vi "Open Sample Container Connections.vi"(8 "error in (no error)":errorcluster, 11 "Sample Line in":refnum<class "Sample Line.lvclass">) -> (0 "error out":errorcluster, 3 "Sample Line out":refnum<class "Sample Line.lvclass">)   [LabVIEW 2015, in "cRIO-Carbondioxide.lvlib" / "CO2-Actor.lvlib" / "Sample Line.lvclass"]
uses:
  Sample Line.lvclass
  Sample Line.lvclass/Sample Line.ctl
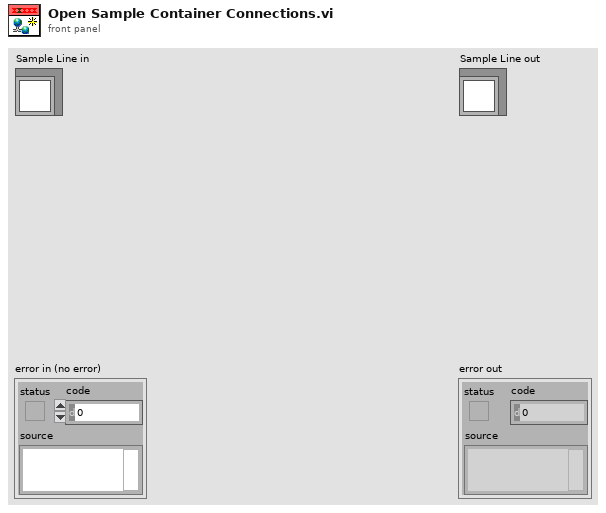
[diagram p1: front panel]
types:
  T1 = typedef "Sample Container.ctl" = cluster{"Sample In":refnum<k21>, "Sample Name":refnum<k21>, "Ti Cathode":refnum<k21>, "SampleQ":refnum<queue>}
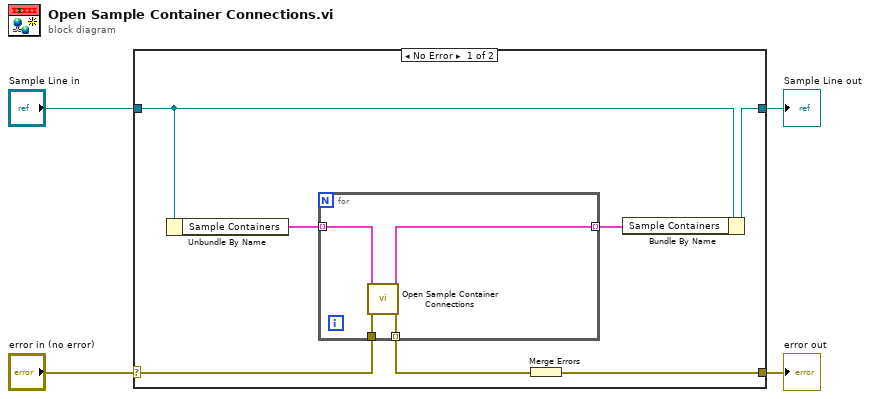
[diagram p0: block diagram]
diagram:
  n1 = case shown="No Error" "error in (no error)" {
    selector: "error in (no error)" -> [w10 w17]
    tunnel: [w8 w17] -> w3
    tunnel: [w5 w16] -> w1
    tunnel: "Sample Line in" -> [w6 w16]
    frame No Error {
      n2 = Unbundle By Name(w6) -> ("Sample Containers"=w11:T1[])
      n3 = for {
        tunnel: w11 -> [w14] mode=indexing
        tunnel: w10 -> [w15]
        tunnel: [w13] -> w7 mode=indexing
        tunnel: [w12] -> w9 mode=indexing
        n4 = call "Open Sample Container Connections.vi"("error in (no error)"=w15, "Container in"=w14) -> ("error out"=w12:errorcluster, "Container out"=w13:T1)  [unwired: 8 in]
      }
      n5 = Merge Errors(w9) -> (w8:errorcluster)
      n6 = Bundle By Name(cluster=w6, "Sample Containers"=w7) -> (w5:refnum<class "Sample Line.lvclass">)
    }
    frame Error {
    }
  }
  "error out" <- w3
  "Sample Line out" <- w1
